vi "UpdateDestroyPositionJustOffset.vi"(0 "Image Settings":T1 {"2nd Axis" items=["x", "y", "z"]; "1st Axis" items=["x", "y", "z"]; "Time Resolution\n(ms/pixel)" format="%.2f"; "Image Resolution (nm/pixel)"."z" format="%.2f"; "Image Resolution (nm/pixel)"."y" format="%.2f"; "Image Resolution (nm/pixel)"."x" format="%.2f"; "Image Size (µm)"."z" format="%.2f"; "Image Size (µm)"."y" format="%.2f"; "Image Size (µm)"."x" format="%.2f"; "End Position (µm)"."z" format="%.2f"; "End Position (µm)"."y" format="%.2f"; "End Position (µm)"."x" format="%.2f"; "Start Position (µm)"."z" format="%.2f"; "Start Position (µm)"."y" format="%.2f"; "Start Position (µm)"."x" format="%.2f"}) -> (1 "error out":errorcluster)   [LabVIEW 2009]
uses:
  ImageSettings.ctt
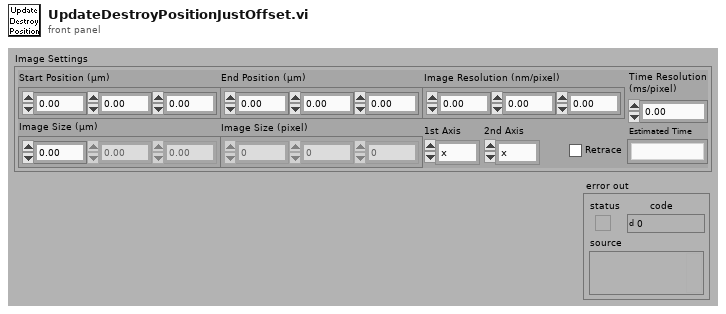
[diagram p1: front panel]
types:
  T1 = typedef "ImageSettings.ctt" = cluster{"Start Position (µm)":cluster{"x":dbl, "y":dbl, "z":dbl}, "End Position (µm)":cluster{"x":dbl, "y":dbl, "z":dbl}, "Image Resolution (nm/pixel)":cluster{"x":dbl, "y":dbl, "z":dbl}, "Image Size (µm)":cluster{"x":dbl, "y":dbl, "z":dbl}, "Image Size (pixel)":cluster{"x":u32, "y":u32, "z":u32}, "Time Resolution\n(ms/pixel)":dbl, "1st Axis":u16, "2nd Axis":u16, "Retrace":bool, "Estimated Time":string}
  T2 = typedef "PickImage.ctl" = cluster{"Rawdata":T3, "Mask":T3, "Display":T3, "Coefficients (2D)":sgl[][], "Destroy Index":u32}
  T3 = typedef "IMAQ Image.ctl" = refnum<image>
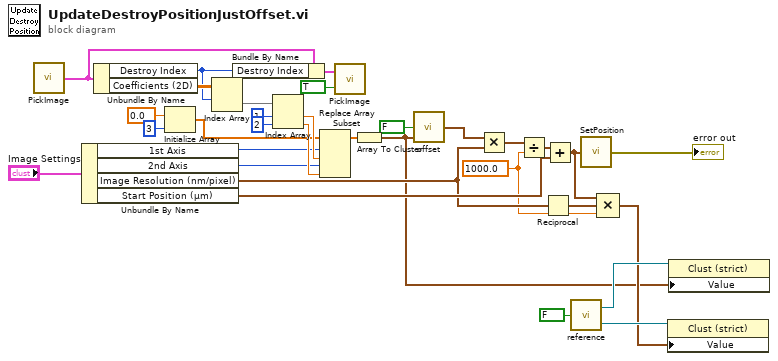
[diagram p0: block diagram]
diagram:
  w10 = 1000.0
  n1 = call "PickImage.vi"() -> ("Image (output)"=w17:T2)  [unwired: 2 in]
  n2 = Unbundle By Name("Image Settings") -> ("1st Axis"=w26:u16, "2nd Axis"=w27:u16, "Image Resolution (nm/pixel)"=w11:cluster{"x":dbl, "y":dbl, "z":dbl}, "Start Position (µm)"=w32:cluster{"x":dbl, "y":dbl, "z":dbl})
  n3 = Unbundle By Name(w17) -> ("Destroy Index"=w1:u32, "Coefficients (2D)"=w18:sgl[][])
  n4 = Initialize Array(0.0 ("element"), 3 ("dimension size")) -> (w25:dbl[])
  n5 = Index Array(array=w18, index (row)=w1) -> (element=w20:sgl[])  [unwired: 1 in]
  n6 = Bundle By Name(cluster=w17, "Destroy Index"=w1) -> (w16:T2)
  n7 = Index Array(array=w20, index #1=1 ("index"), index #2=2 ("index")) -> (element #1=w29:sgl, element #2=w30:sgl)
  n8 = Replace Array Subset(array=w25, new element #1=w29, index #1=w26, new element #2=w30, index #2=w27) -> (w28:dbl[])
  n9 = call "PickImage.vi"("Get/Set"=TRUE, "Images (input)"=w16) -> ()  [unwired: 1 out]
  n10 = Array To Cluster(array=w28) -> (cluster=w2:cluster{"[0]":dbl, "[1]":dbl, "[2]":dbl})
  n11 = call "offset.vi"("coordinates (in)"=w2, "set?"=FALSE) -> ("coordinates (out)"=w8:cluster{dbl, dbl, dbl})  [unwired: 1 in]
  n12 = Multiply(x=w8, y=w11) -> (x*y=w31:cluster{dbl, dbl, dbl})
  n13 = Divide(x=w31, y=w10) -> (x/y=w14:cluster{dbl, dbl, dbl})
  n14 = Reciprocal(x=w11) -> (1/x=w9:cluster{"x":dbl, "y":dbl, "z":dbl})
  n15 = Add(x=w14, y=w32) -> (x+y=w12:cluster{dbl, dbl, dbl})
  n16 = call "reference.vi"("set?"=FALSE) -> ("coordinates (pixel) 2"=w5:refnum<vi>, "Pickcoord. (pixel) 2"=w4:refnum<vi>)  [unwired: 3 in]
  n17 = call "SetPosition.vi"("Current Position (µm)"=w12) -> ("error out"=→"error out":errorcluster)
  n18 = Compound Arithmetic op=MULTIPLY(w12, w9, w10) -> (w3:cluster{dbl, dbl, dbl})
  n19 = property class="Clust (strict)"(reference=w5, "Value"=w3) -> ()  [unwired: 1 in, 2 out]
  n20 = property class="Clust (strict)"(reference=w4, "Value"=w2) -> ()  [unwired: 1 in, 2 out]
